vi "ManualL1Control.vi"() -> ()   [LabVIEW 2012]
uses:
  <vilib>/Utility/NIReport.llb/NI_report.lvclass
  <vilib>/Utility/NIReport.llb/HTML/NI_HTML.lvclass
panel:
  in  "Adder B0":u32=25 max=255 step=1
  in  "Adder B1":u32=255 max=255 step=1
  in  "Adder C0":u32=255 max=255 step=1
  in  "Adder C1":u32=255 max=255 step=1
  in  "Adder A0":u32=255 max=255 step=1
  in  "Adder A1":u32=255 max=255 step=1
  in  "Adder B 1":u32(slide)=255 max=255 step=1 scale=0.0..255.0
  in  "Adder A 1":u32(slide)=255 max=255 step=1 scale=0.0..255.0
  in  "Adder C 1":u32(slide)=255 max=255 step=1 scale=0.0..255.0
  out "Data out 0":string="empty_read_buffer0_2-65@1\r\n0_2-68@1\r\n"
  out "IPR value 0":i32=1
  out "hex 7":string="3400"
  out "hex 6":string="7BF"
  out "hex 5":string="FFFF"
  out "hex 4":string="19FF"
  out "hex 3":string="FFFF"
  out "hex 2":string="FFFF"
  out "hex":string="2AAA"
  out "Data out 1":string="empty_read_buffer0_2-65@1\r\n0_2-69@0\r\n"
  out "IPR value 1":i32
  in  "Adder B 0":u32(slide) max=255 step=1 scale=0.0..255.0
  in  "Adder A 0":u32(slide)=255 max=255 step=1 scale=0.0..255.0
  in  "Adder C 0":u32(slide)=255 max=255 step=1 scale=0.0..255.0
  in  "stop":bool
  in  "Instrument VISA in":T1={"AWG VISA"="AgilentGenerator1", "Oscilloscope  VISA "="AgilentOsciloscope", "Integration Board IP"="172.16.17.47", "connection ID"=refnum, "report out"=refnum, "report file path"=path "C:/Documents and Settings/CTA_LAB01/Desktop/L0_Asic/L0 Asic Test Data"}
  in  "SingleIN/#Combination":bool=TRUE
  in  "Combination":i32 min=0 max=127 step=1 format="%b"
  in  "! All Channels \n(false activates all channels)":bool=TRUE
  in  "Enable  L1 single  Input":i32(slide) scale=0.0..6.0
  in  "error in":errorcluster
  out "data out serial":string="empty_read_bufferwrittingempty_read_bufferwritting2"
  out "error out":errorcluster
  out "REG Array":u32[](array[numeric])=[10922, 65535, 65535, 6655, 65535, 1983, 13312]
  in  "Register Adress 96":bool[](array[boolean])=[FALSE, TRUE, FALSE, TRUE, FALSE, TRUE, FALSE, TRUE, FALSE, TRUE, FALSE, TRUE, FALSE, TRUE, FALSE, FALSE]
  out "REG 96":u32=10922
  out "?":bool[](array[boolean])=[TRUE, TRUE, TRUE, TRUE, TRUE, TRUE, TRUE, TRUE, TRUE, FALSE, FALSE, TRUE, TRUE, FALSE, FALSE, FALSE, FALSE, FALSE, FALSE, FALSE, FALSE, FALSE, FALSE, FALSE, FALSE, FALSE, FALSE, FALSE, FALSE, FALSE, FALSE, FALSE, FALSE, FALSE, FALSE, FALSE, FALSE, FALSE, FALSE, FALSE, FALSE, FALSE, FALSE, FALSE, FALSE, FALSE, FALSE, FALSE, FALSE, FALSE, FALSE, FALSE, FALSE, FALSE, FALSE, FALSE, FALSE, FALSE, FALSE, FALSE, FALSE, FALSE, FALSE, FALSE]
  out "REG 99":u32=6655
  out "?":bool[](array[boolean])=[TRUE, TRUE, TRUE, TRUE, TRUE, TRUE, TRUE, TRUE, TRUE, TRUE, TRUE, TRUE, TRUE, TRUE, TRUE, TRUE, FALSE, FALSE, FALSE, FALSE, FALSE, FALSE, FALSE, FALSE, FALSE, FALSE, FALSE, FALSE, FALSE, FALSE, FALSE, FALSE, FALSE, FALSE, FALSE, FALSE, FALSE, FALSE, FALSE, FALSE, FALSE, FALSE, FALSE, FALSE, FALSE, FALSE, FALSE, FALSE, FALSE, FALSE, FALSE, FALSE, FALSE, FALSE, FALSE, FALSE, FALSE, FALSE, FALSE, FALSE, FALSE, FALSE, FALSE, FALSE]
  out "REG 98":u32=65535
  out "?":bool[](array[boolean])=[TRUE, TRUE, TRUE, TRUE, TRUE, TRUE, TRUE, TRUE, TRUE, TRUE, TRUE, TRUE, TRUE, TRUE, TRUE, TRUE, FALSE, FALSE, FALSE, FALSE, FALSE, FALSE, FALSE, FALSE, FALSE, FALSE, FALSE, FALSE, FALSE, FALSE, FALSE, FALSE, FALSE, FALSE, FALSE, FALSE, FALSE, FALSE, FALSE, FALSE, FALSE, FALSE, FALSE, FALSE, FALSE, FALSE, FALSE, FALSE, FALSE, FALSE, FALSE, FALSE, FALSE, FALSE, FALSE, FALSE, FALSE, FALSE, FALSE, FALSE, FALSE, FALSE, FALSE, FALSE]
  out "REG 97":u32=65535
  in  "Register Adress 102":bool[](array[boolean])=[FALSE, FALSE, FALSE, FALSE, FALSE, FALSE, FALSE, FALSE, FALSE, FALSE, TRUE, FALSE, TRUE, TRUE, FALSE, FALSE]
  out "REG 102":u32=13312
  in  "Register Adress 101":bool[](array[boolean])=[TRUE, TRUE, TRUE, TRUE, TRUE, TRUE, FALSE, TRUE, TRUE, TRUE, TRUE, FALSE, FALSE, FALSE, FALSE, FALSE]
  out "REG 101":u32=1983
  in  "Register Adress 100":bool[](array[boolean])=[TRUE, TRUE, TRUE, TRUE, TRUE, TRUE, TRUE, TRUE, TRUE, TRUE, TRUE, TRUE, TRUE, TRUE, TRUE, TRUE]
  out "REG 100":u32=65535
  # "0           1            2"
  # "DAC_TH0"
  # "DAC_TH1"
  # "DAC_TH2"
  # "DAC_TH3"
  # "DAC_TH4"
  # "DAC_TH5"
  # "Unused"
  # "DAC_MUX_ENA"
  # "ADDER_C"
  # "LSB"
  # "MSB"
  # "ADDER_A"
  # "LSB"
  # "MSB"
  # "ADDER_B"
  # "LSB"
  # "MSB"
  # "a         b         c"
  # "a         b         c"
  # "a         b         c"
  # "a         b         c"
  # "a         b         c"
  # "Unused"
  # "CH0"
  # "CH1"
  # "CH2"
  # "CH3"
  # "CH4"
  # "a         b         c"
  # "ENA_0  ENA_1"
  # "ENA_0  ENA_1"
  # "a         b         c"
  # "BUFF\nENA"
  # "R       E       S      E        R     V        E      D"
  # "CH5"
  # "CH6"
  # "MUX"
  # "LVDS"
  # "R               E               S               E                  R                V             E              D"
  # "0            1            2            3           4             5"
  # "DAC _IB"
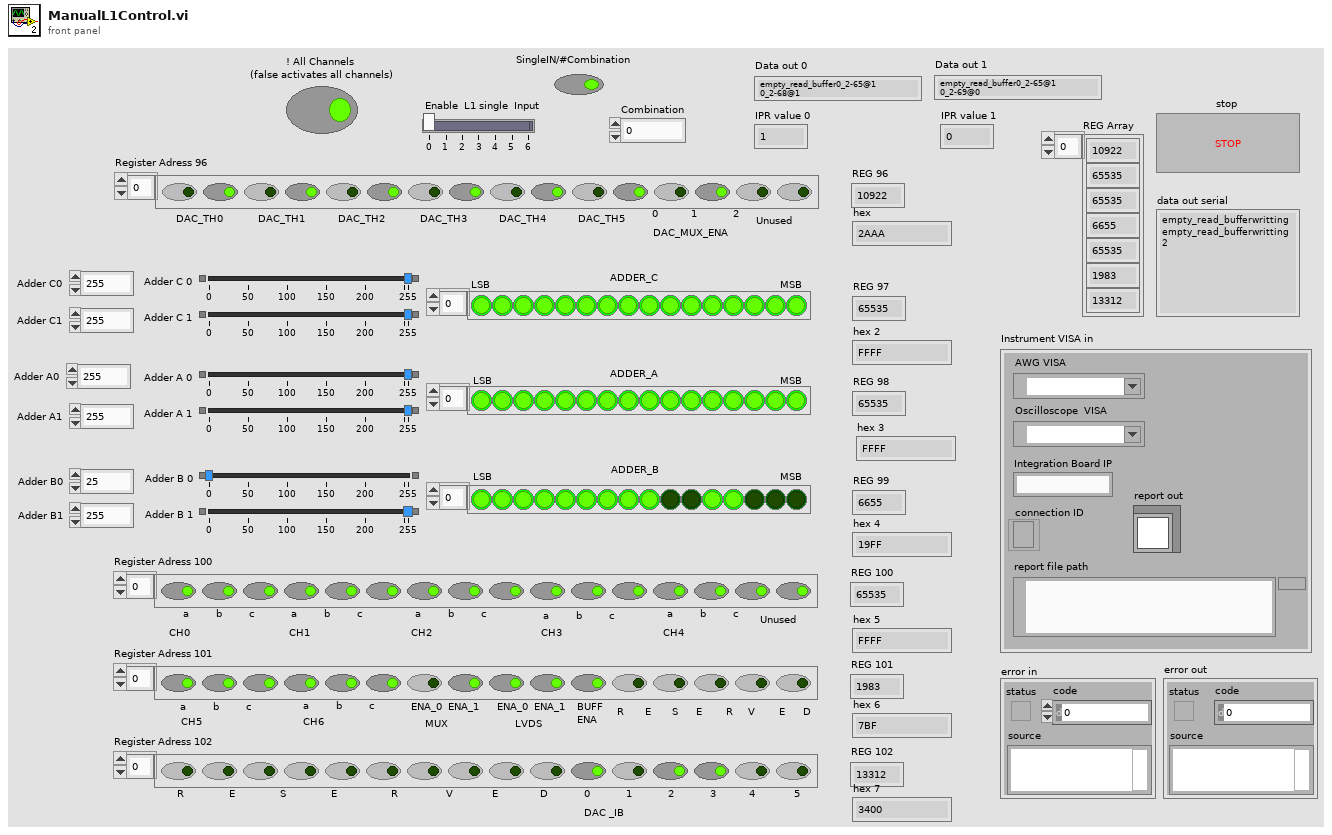
[diagram p1: front panel]
types:
  T1 = cluster{"AWG VISA":refnum<visa-resource-name>, "Oscilloscope  VISA ":refnum<visa-resource-name>, "Integration Board IP":string, "connection ID":refnum<k5>, "report out":refnum<class "NI_report.lvclass">, "report file path":path}
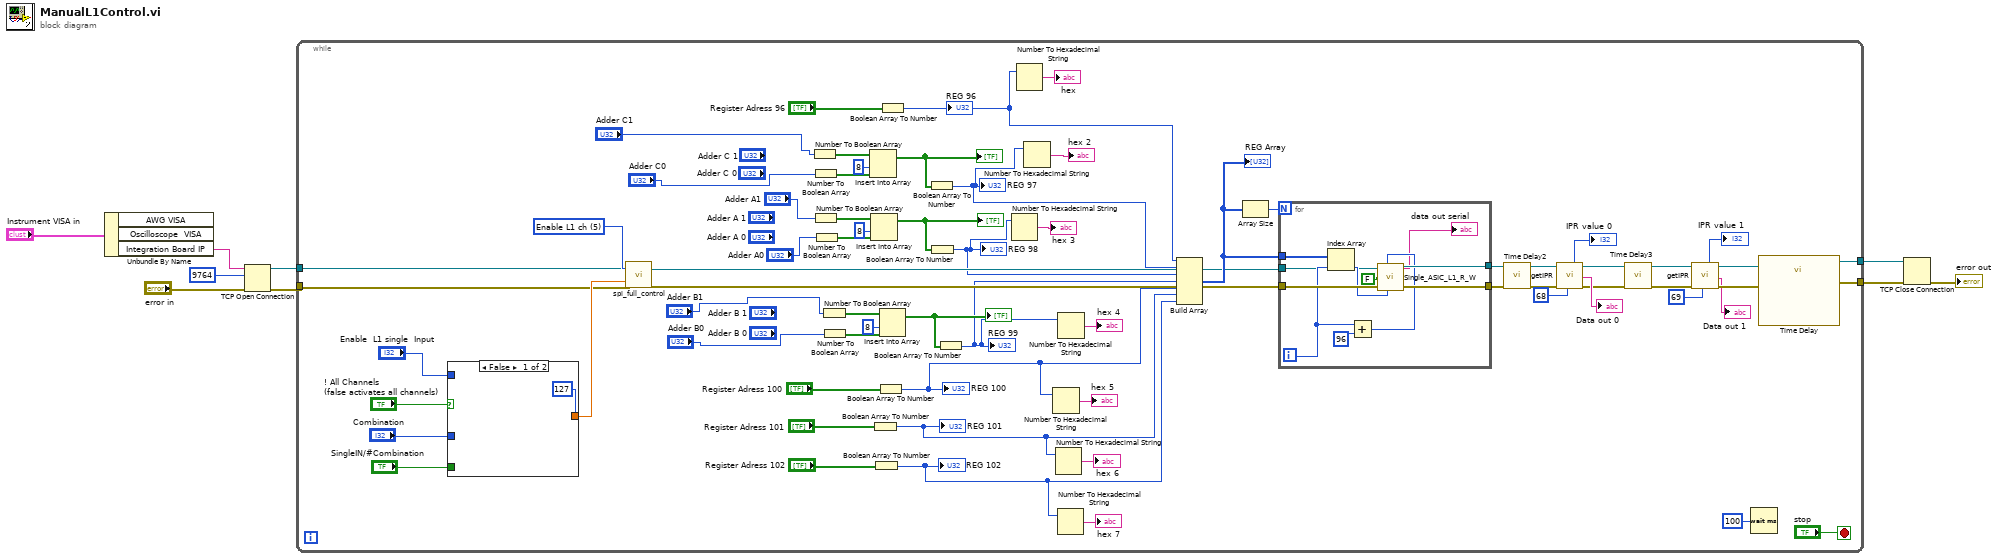
[diagram p0: block diagram]
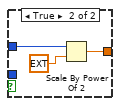
[diagram p3: hidden frame]
diagram:
  n1 = Unbundle By Name("Instrument VISA in") -> ("Integration Board IP"=w8:string)  [unwired: 2 out]
  n2 = TCP Open Connection(address=w8, remote port or service name=9764, error in (no error)="error in") -> (connection ID=w4:refnum<k5>, error out=w3:errorcluster)  [unwired: 2 in]
  n3 = while {
    tunnel: w4 -> [w48]
    tunnel: w3 -> [w47]
    tunnel: [w44] -> w2
    tunnel: [w26] -> w1
    stop <- "stop" stop-if-true
    w54 = u16 5 items=["Attenuation", "Clipping", "Enable channel", "Delay line", "ASIC", "Enable L1 ch", "ASIC L1"] ("Device")
    n4 = case shown="False" "! All Channels \n(false activates all channels)" {
      tunnel: [127 ("Register or channel") w78] -> w55
      tunnel: "Enable  L1 single  Input" -> [_ w79]
      tunnel: "Combination" -> [_ w77]
      tunnel: "SingleIN/#Combination" -> [_ w76]
      frame False {
      }
      frame True {
        n5 = case shown="False" w76 {
          tunnel: w79 -> [_ w82]
          tunnel: [w80 w81] -> w78
          tunnel: w77 -> [w80 _]
          frame False {
          }
          frame True {
            n6 = Scale By Power Of 2(n=w82, x=ext 1.0) -> (x*2^n=w81:ext)
          }
        }
      }
    }
    n7 = call "spi_full_control.vi"("connection ID"=w48, "Device"=w54, "Data"=w55, "error out 3"=w47) -> ("connection ID out"=w49:refnum<k5>, "error out 2"=w50:errorcluster)  [unwired: 8 in, 6 out]
    n8 = Number To Boolean Array(number="Adder C1") -> (Boolean array=w71:bool[])
    n9 = Number To Boolean Array(number="Adder C0") -> (Boolean array=w70:bool[])
    n10 = Number To Boolean Array(number="Adder A1") -> (Boolean array=w67:bool[])
    n11 = Number To Boolean Array(number="Adder A0") -> (Boolean array=w66:bool[])
    n12 = Number To Boolean Array(number="Adder B1") -> (Boolean array=w63:bool[])
    n13 = Number To Boolean Array(number="Adder B0") -> (Boolean array=w62:bool[])
    n14 = Insert Into Array(array=w71, index=8, new element=w70) -> (w69:bool[])
    "?" <- w69
    n15 = Insert Into Array(array=w67, index=8, new element=w66) -> (w65:bool[])
    "?" <- w65
    n16 = Boolean Array To Number(Boolean array="Register Adress 101") -> (number=w32:u32)
    "REG 101" <- w32
    n17 = Boolean Array To Number(Boolean array="Register Adress 102") -> (number=w30:u32)
    "REG 102" <- w30
    n18 = Boolean Array To Number(Boolean array="Register Adress 100") -> (number=w34:u32)
    "REG 100" <- w34
    n19 = Insert Into Array(array=w63, index=8, new element=w62) -> (w61:bool[])
    "?" <- w61
    n20 = Boolean Array To Number(Boolean array="Register Adress 96") -> (number=w42:u32)
    "REG 96" <- w42
    n21 = Boolean Array To Number(Boolean array=w69) -> (number=w39:u32)
    "REG 97" <- w39
    n22 = Boolean Array To Number(Boolean array=w65) -> (number=w38:u32)
    "REG 98" <- w38
    n23 = Boolean Array To Number(Boolean array=w61) -> (number=w36:u32)
    "REG 99" <- w36
    n24 = Number To Hexadecimal String(2:w38) -> (0:→"hex 3":string)  [unwired: 1 in]
    n25 = Number To Hexadecimal String(2:w42) -> (0:→"hex":string)  [unwired: 1 in]
    n26 = Number To Hexadecimal String(2:w39) -> (0:→"hex 2":string)  [unwired: 1 in]
    n27 = Number To Hexadecimal String(2:w34) -> (0:→"hex 5":string)  [unwired: 1 in]
    n28 = Number To Hexadecimal String(2:w32) -> (0:→"hex 6":string)  [unwired: 1 in]
    n29 = Number To Hexadecimal String(2:w30) -> (0:→"hex 7":string)  [unwired: 1 in]
    n30 = Number To Hexadecimal String(2:w36) -> (0:→"hex 4":string)  [unwired: 1 in]
    n31 = Build Array(w42, w39, w38, w36, w34, w32, w30) -> (w57:u32[])
    "REG Array" <- w57
    n32 = Array Size(array=w57) -> (size(s)=w58:i32)
    n33 = for {
      N: w58 -> [_]
      tunnel: w50 -> [w94]
      tunnel: w57 -> [w93]
      tunnel: [w92] -> w19
      tunnel: [w91] -> w21
      tunnel: w49 -> [w84]
      i -> [w87]
      n34 = Index Array(array=w93, index=w87) -> (element=w90:u32)
      n35 = Add(x=w87, y=96) -> (x+y=w88:i32)
      n36 = call "Single_ASIC_L1_R_W.vi"("connection ID"=w84, "Register or channel"=w88, "RD/#WR"=FALSE, "error in (no error)"=w94, "Data"=w90) -> ("data out serial"=→"data out serial":string, "connection ID out"=w92:refnum<k5>, "error out"=w91:errorcluster)  [unwired: 1 in, 1 out]
    }
    n37 = call "Time Delay2"("error in (no error)"=w21) -> ("error out"=w17:errorcluster)  [unwired: 10 in]
    n38 = call "getIPR.vi"("Address"=68, "error in"=w17, "connection ID"=w19) -> ("error out"=w20:errorcluster, "Data"=→"Data out 0":string, "connection ID out"=w18:refnum<k5>, "IPR_count"=→"IPR value 0":u32)  [unwired: 5 in]
    n39 = call "Time Delay3"("error in (no error)"=w20) -> ("error out"=w16:errorcluster)  [unwired: 10 in]
    n40 = call "getIPR.vi"("Address"=69, "error in"=w16, "connection ID"=w18) -> ("error out"=w29:errorcluster, "Data"=→"Data out 1":string, "connection ID out"=w26:refnum<k5>, "IPR_count"=→"IPR value 1":u32)  [unwired: 5 in]
    n41 = Wait (ms)(milliseconds to wait=u32 100) -> ()  [unwired: 1 out]
    n42 = call "Time Delay"("error in (no error)"=w29) -> ("error out"=w44:errorcluster)  [unwired: 10 in]
  }
  n43 = TCP Close Connection(connection ID=w1, error in (no error)=w2) -> (error out=→"error out":errorcluster)  [unwired: 1 in, 1 out]
